vi "plot_loadDisdrometer.vi"(0 "Output Path":path=path "C:/Disdrometer/Data", 2 "File Prefix":string="Disdrometer", 9 "Time":timestamp, 11 "Offset (hrs)":dbl) -> (8 "Loaded Data Array":dbl[][](array[numeric]), 15 "Timestamp":dbl[](array[numeric]))   [LabVIEW 2018]
uses:
  <vilib>/Utility/file.llb/Read From Spreadsheet File (DBL).vi
panel:
  out "Rain Accum":dbl[](array[numeric])
  out "Rain Rate":dbl[](array[numeric])
  out "Timestamp":dbl[](array[numeric])
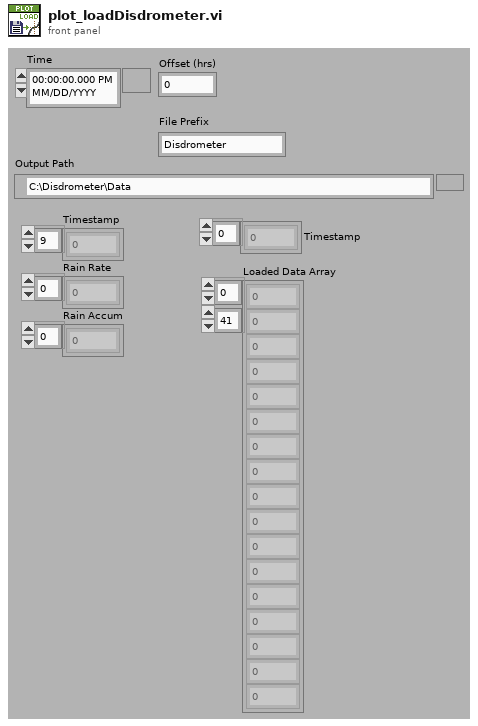
[diagram p1: front panel]
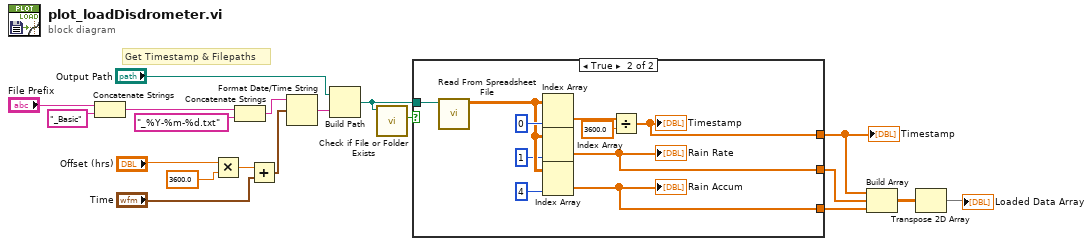
[diagram p0: block diagram]
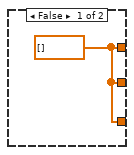
[diagram p2: hidden frame]
diagram:
  # "Get Timestamp & Filepaths"
  n1 = Concatenate Strings("File Prefix", "_Basic" ("string")) -> (w1:string)
  n2 = Multiply(x="Offset (hrs)", y=3600.0) -> (x*y=w18:dbl)
  n3 = Concatenate Strings(w1, "_%Y-%m-%d.txt" ("string")) -> (w16:string)
  n4 = Add(x=w18, y="Time") -> (x+y=w10:timestamp)
  n5 = Format Date/Time String(time format string (%c)=w16, seconds (now)=w10) -> (date/time string=w17:string)  [unwired: 1 in]
  n6 = Build Path(base path="Output Path", name or relative path=w17) -> (appended path=w13:path)
  n7 = call <vilib>:"Check if File or Folder Exists.vi"("path"=w13) -> ("file or folder exists?"=w12:bool)  [unwired: 8 in, 2 out]
  n8 = case shown="True" w12 {
    tunnel: w13 -> [_ w26]
    tunnel: [w20 w21] -> w6
    tunnel: [w20 w25] -> w5
    tunnel: [w20 w24] -> w4
    frame False {
      w20 = dbl[] [] ("all rows")
    }
    frame True {
      n9 = call-poly <vilib>:"Read From Spreadsheet File.vi"("file path (dialog if empty)"=w26) -> ("all rows"=w29:dbl[][])  [unwired: 6 in, 4 out]
      n10 = Index Array(array=w29, index (col)=0 ("disabled index (col)")) -> (element=w22:dbl[])  [unwired: 1 in]
      n11 = Index Array(array=w29, index (col)=1 ("disabled index (col)")) -> (element=w25:dbl[])  [unwired: 1 in]
      "Rain Rate" <- w25
      n12 = Index Array(array=w29, index (col)=4 ("disabled index (col)")) -> (element=w24:dbl[])  [unwired: 1 in]
      "Rain Accum" <- w24
      n13 = Divide(x=w22, y=3600.0) -> (x/y=w21:dbl[])
      "Timestamp" <- w21
    }
  }
  "Timestamp" <- w6
  n14 = Build Array(w6, w5, w4) -> (w7:dbl[][])
  n15 = Transpose 2D Array(2D array=w7) -> (transposed array=→"Loaded Data Array":dbl[][])
